vi "AK TCP Factory.vi"(8 "error in (no error)":errorcluster, 10 "AK TCP settings":T1) -> (0 "error out":errorcluster, 3 "protocol out":refnum<class "Protocol Parent.lvclass">)   [LabVIEW 2023, in "Protocols.lvlib" / "AK TCP.lvclass"]
doc: "Instantiates a new AK TCP Protocol object using the provided AK TCP settings."
uses:
  AK TCP.lvclass
  Protocol Parent/Protocol Parent.lvclass
  AK TCP Settings.ctl
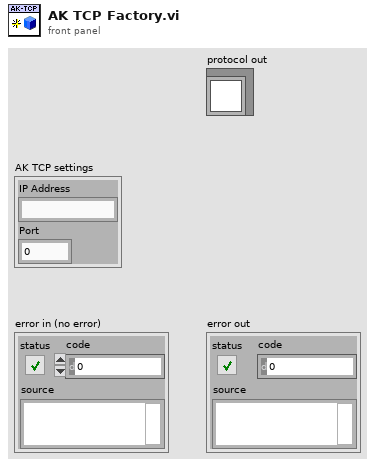
[diagram p1: front panel]
types:
  T1 = typedef "Protocols.lvlib/AK TCP.lvclass/AK TCP Settings.ctl" = cluster{"IP Address":string, "Port":u16}
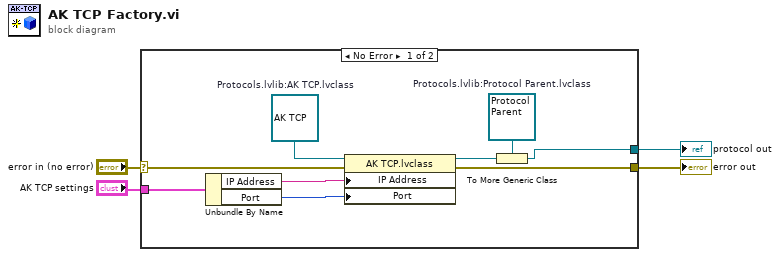
[diagram p0: block diagram]
diagram:
  n1 = case shown="No Error" "error in (no error)" {
    selector: "error in (no error)" -> [w8 w14]
    tunnel: "AK TCP settings" -> [w12 _]
    tunnel: [w9 w14] -> w3
    tunnel: [w5 _] -> w1
    frame No Error {
      w6 = refnum<class "Protocol Parent.lvclass"> refnum  # Protocols.lvlib:Protocol Parent.lvclass
      w13 = refnum<class "AK TCP.lvclass"> refnum  # Protocols.lvlib:AK TCP.lvclass
      n2 = Unbundle By Name(w12) -> ("IP Address"=w11:string, "Port"=w10:u16)
      n3 = property class="AK TCP.lvclass"(reference=w13, error in=w8, "IP Address"=w11, "Port"=w10) -> (reference out=w7:refnum<class "AK TCP.lvclass">, error out=w9:errorcluster)
      n4 = To More Generic Class(target class=w6, reference=w7) -> (generic class reference=w5:refnum<class "Protocol Parent.lvclass">)
    }
    frame Error {
    }
  }
  "error out" <- w3
  "protocol out" <- w1
